vi "AutoSchedule.vi"() -> ()   [LabVIEW 2012]
uses:
  <vilib>/Utility/NIReport.llb/NI_report.lvclass
  <vilib>/addons/database/Auxilliary.llb/DB Tools Cursor Type.ctl
  <vilib>/addons/_office/_exclsub.llb/font.ctl
  <vilib>/addons/_office/excel.llb/Excel Get Data (str).vi
  <vilib>/addons/database/Connection.llb/DB Tools Open Connec (Path).vi
  <vilib>/addons/database/Connection.llb/Conn Execute.vi
  <vilib>/addons/database/Recordset.llb/Rec Fetch Recordset Data (R).vi
  <vilib>/addons/database/Recordset.llb/Rec Destroy - Connection.vi
  <vilib>/Utility/NIReport.llb/Excel/NI_Excel.lvclass
  <vilib>/addons/_office/NI_ReportGenerationToolkit.lvlib
  <vilib>/addons/database/NI_Database_API.lvlib
panel:
  out "error out":errorcluster
  out "concatenated string 2":string
  out "error out 5":errorcluster
  in  "start (0, 0) 4":cluster{"start row":i32, "start column":i32}
  out "concatenated string":string
  in  "start (0, 0) 3":cluster{"start row":i32, "start column":i32}
  out "Numeric":i32
  out "ExcelRow":i32
  in  "start (0, 0)":cluster{"start row":i32, "start column":i32}
  out "x+y":i32
  in  "start (0, 0) 2":cluster{"start row":i32, "start column":i32}
  out "row":i32
  out "array":string[][](array[string])
  out "error out 4":errorcluster
  out "spreadsheet string":string
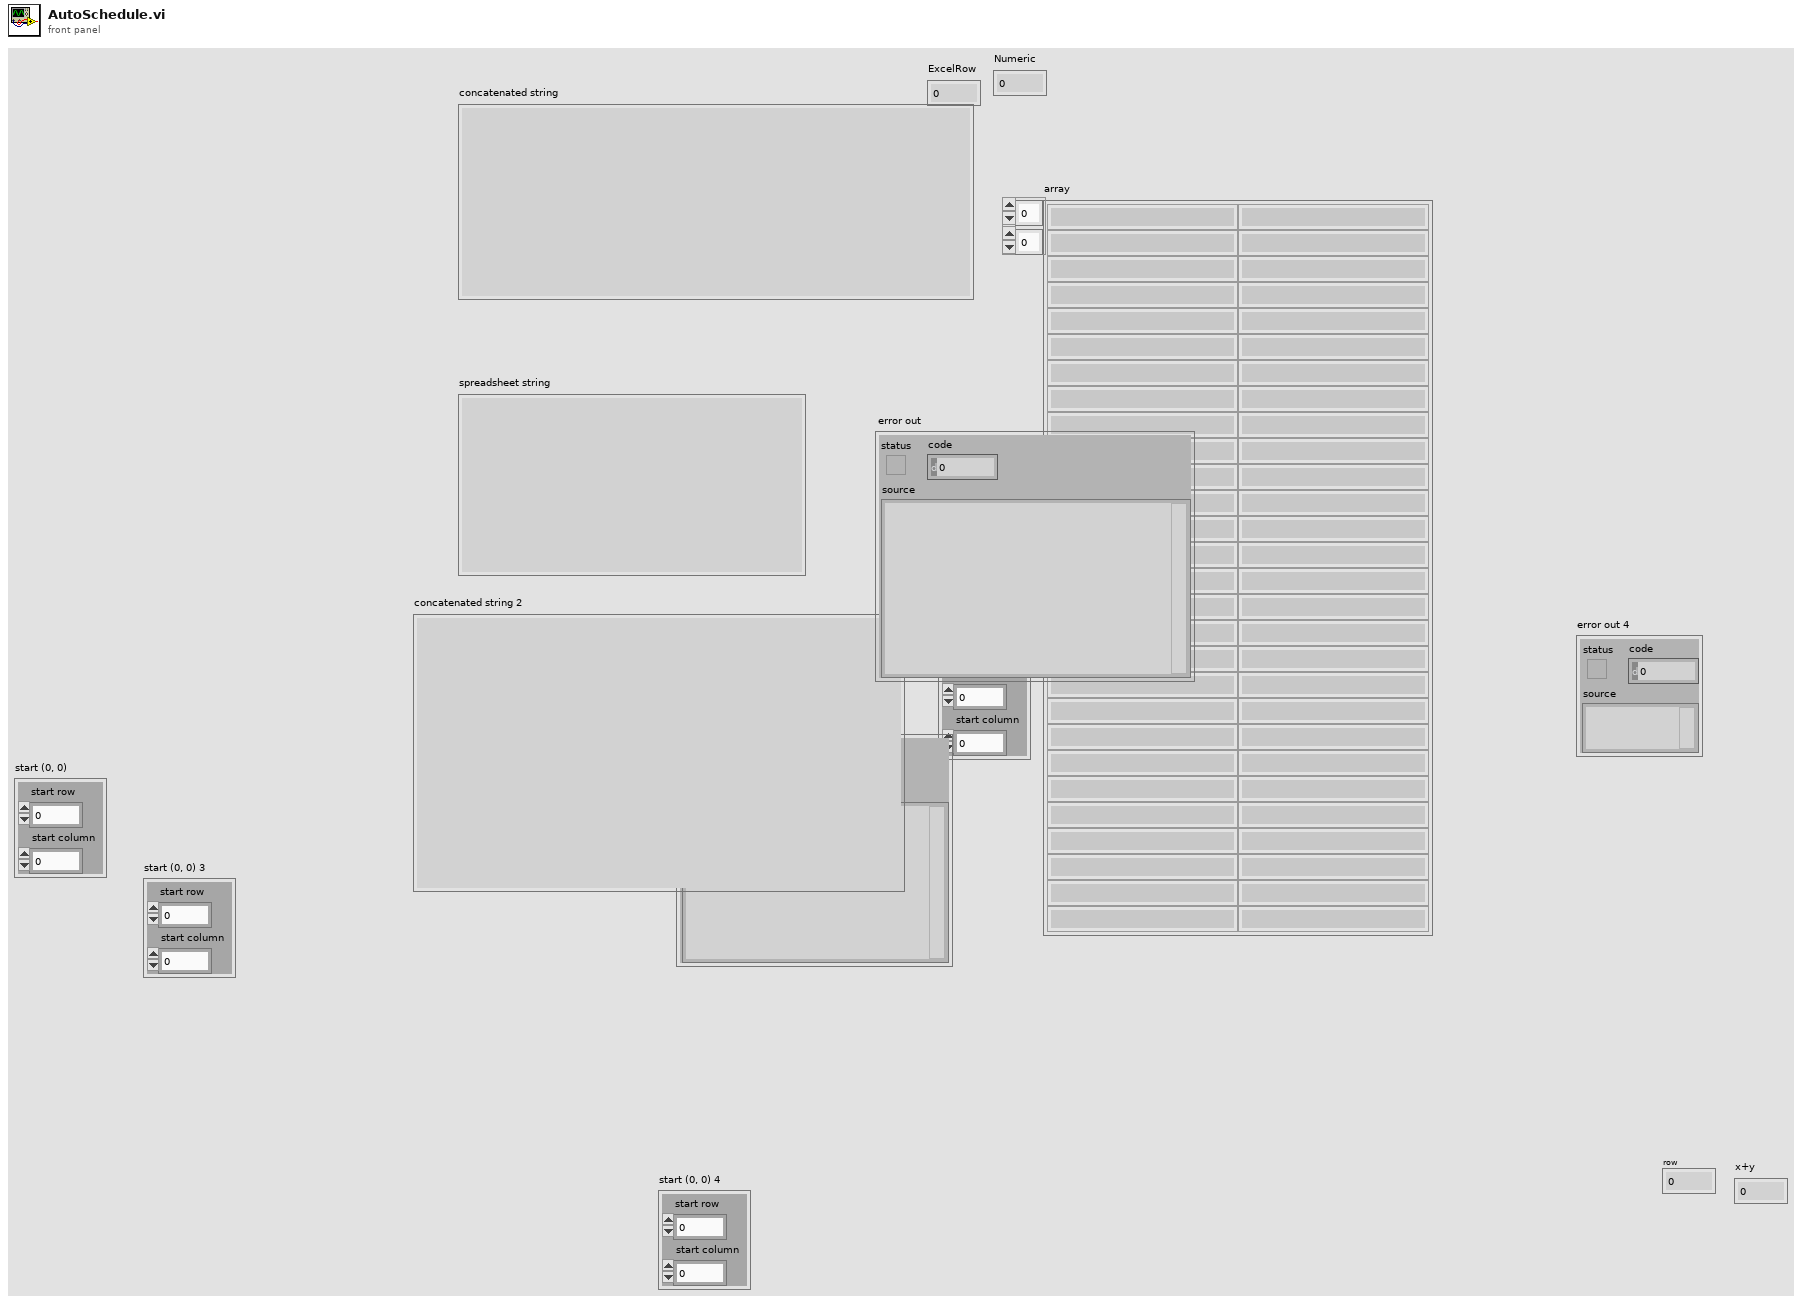
[diagram p1: front panel]
types:
  T1 = enum16{"Standard Report", "HTML", "Word", "Excel"}
  T2 = typedef "NI_ReportGenerationToolkit.lvlib/font.ctl" = cluster{"font name":string, "font size":dbl, "bold":u16, "italic":u16, "underline":u16, "strike through":u16, "font color":u32}
  T3 = cluster{"on/off":bool, "weight":i32, "color":u32}
  T4 = typedef "NI_Database_API.lvlib/DB Tools Cursor Type.ctl" = enum16{"forward-only", "keyset", "dynamic", "static"}
  T5 = typedef "NI_Database_API.lvlib/Conn ObjectReference.ctl" = refnum<k1>
  T6 = typedef "NI_Database_API.lvlib/Rec ObjectReference.ctl" = refnum<k1>
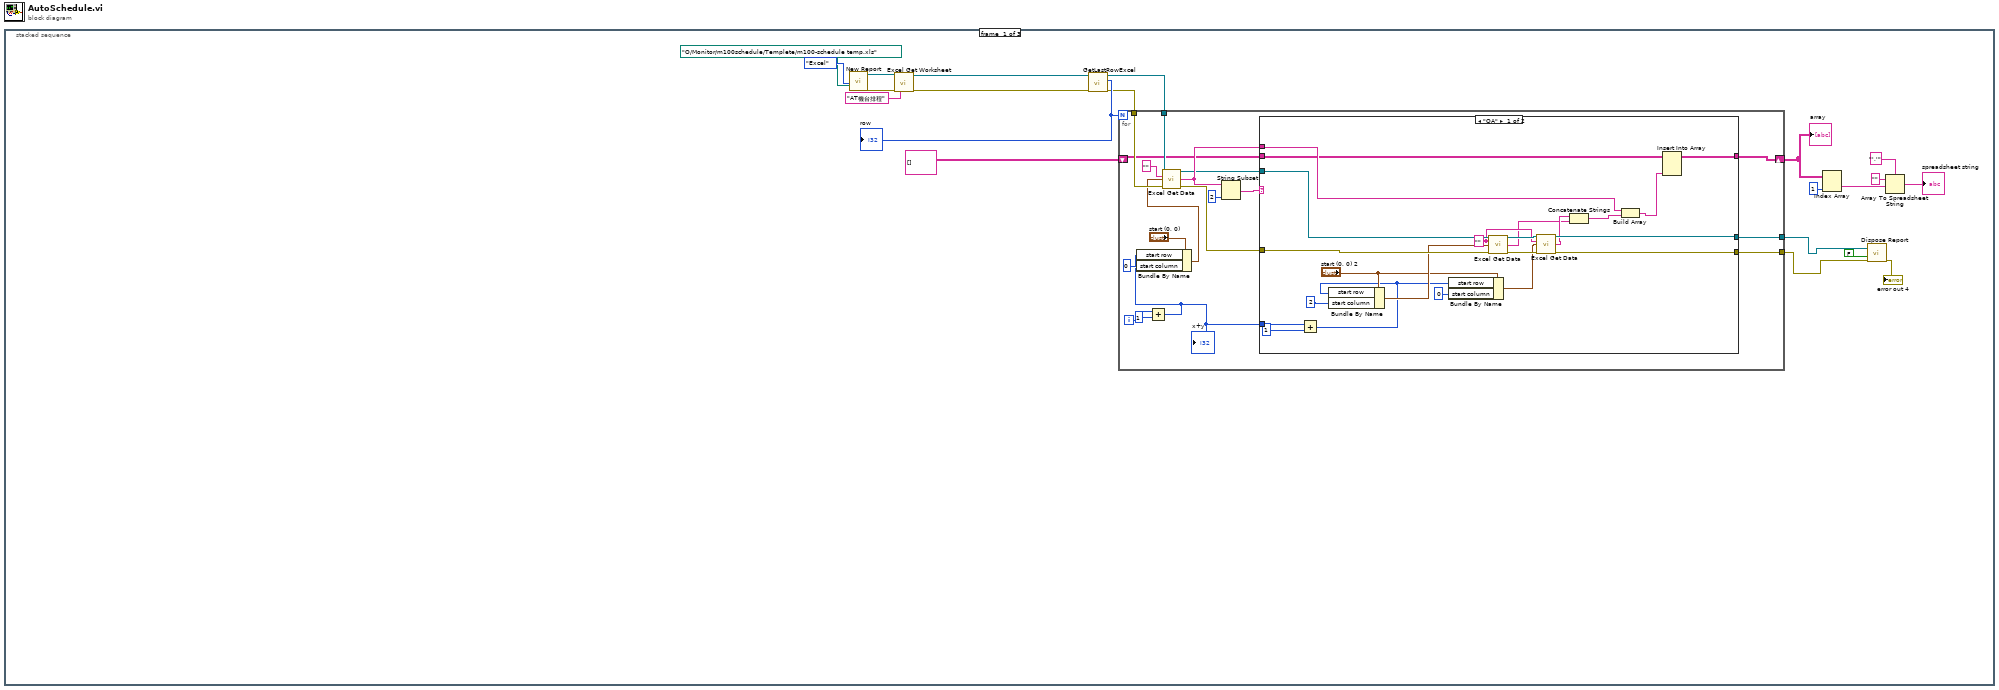
[diagram p0: block diagram]
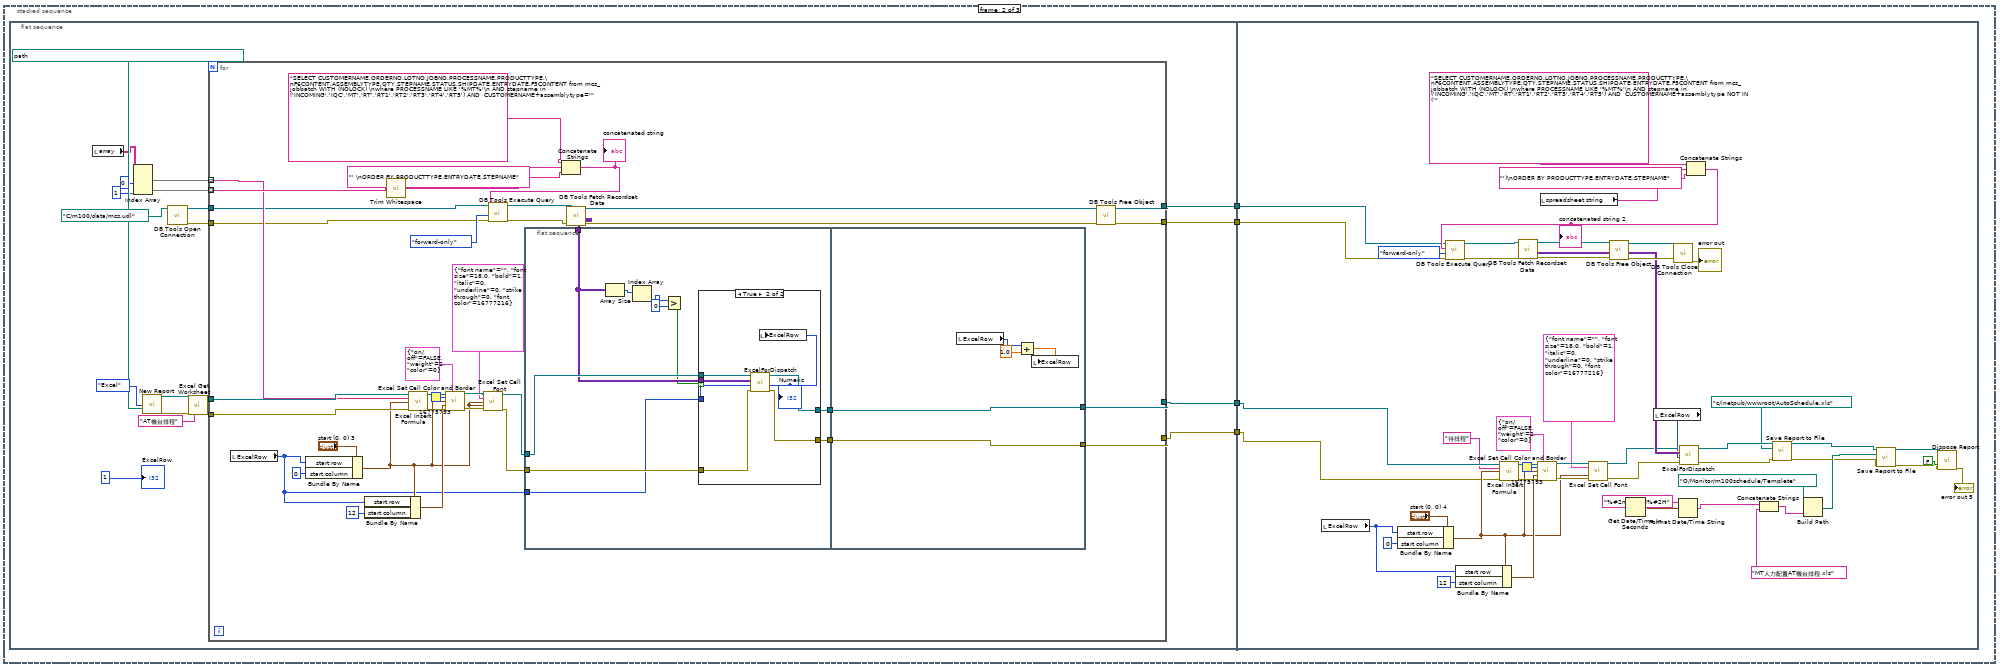
[diagram p3: hidden frame]
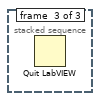
[diagram p5: hidden frame]
diagram:
  n1 = stacked-sequence {
    frame #0 {
      n2 = call <vilib>:"New Report.vi"("report type"=T1."Excel" ("Report Type"), "template (empty)"=path "O:/Monitor/m100schedule/Templete/m100-schedule temp.xls") -> ("report out"=w20:refnum<class "NI_report.lvclass">, "error out"=w19:errorcluster)  [unwired: 12 in]
      n3 = call <vilib>:"Excel Get Worksheet.vi"("report in"=w20, "error in (no error)"=w19, "name (\"\")"="AT機台排程" ("name (\"\")")) -> ("report out"=w18:refnum<class "NI_report.lvclass">, "error out"=w17:errorcluster)  [unwired: 11 in]
      n4 = call "GetLastRowExcel.vi"("error in (no error)"=w17, "report in"=w18) -> ("error out"=w13:errorcluster, "row"=w16:i32, "report out"=w12:refnum<class "NI_report.lvclass">)  [unwired: 7 in]
      "row" <- w16
      n5 = for {
        N: w16 -> [_]
        tunnel: w12 -> [w39]
        tunnel: w13 -> [w38]
        shift-right: [w27] -> w3
        shift-left: string[][] [] ("array") -> [w28]
        tunnel: [w23] -> w8
        tunnel: [w22] -> w7
        i -> [w34]
        n6 = Add(x=w34, y=1) -> (x+y=w24:i32)
        "x+y" <- w24
        n7 = Bundle By Name(cluster="start (0, 0)", "start row"=w24, "start column"=0) -> (w35:cluster{"start row":i32, "start column":i32})
        n8 = call-poly <vilib>:"Excel Get Data.vi"("report in"=w39, "data type"="", "start (0, 0)"=w35, "error in (no error)"=w38) -> ("report out"=w26:refnum<class "NI_report.lvclass">, "data"=w30:string, "error out"=w25:errorcluster)  [unwired: 9 in]
        n9 = String Subset(string=w30, length (rest)=2 ("length (rest)")) -> (substring=w31:string)  [unwired: 1 in]
        n10 = case shown="\"QA\"" w31 {
          tunnel: w30 -> [w61 _]
          tunnel: w28 -> [w58 w64]
          tunnel: [w59 w64] -> w27
          tunnel: w26 -> [w57 w63]
          tunnel: w25 -> [w56 w62]
          tunnel: w24 -> [w53 _]
          tunnel: [w50 w63] -> w23
          tunnel: [w48 w62] -> w22
          frame "QA" {
            w47 = "" ("data type")
            n11 = Add(x=w53, y=1) -> (x+y=w44:i32)
            n12 = Bundle By Name(cluster="start (0, 0) 2", "start row"=w44, "start column"=2) -> (w55:cluster{"start row":i32, "start column":i32})
            n13 = Bundle By Name(cluster="start (0, 0) 2", "start row"=w44, "start column"=0) -> (w46:cluster{"start row":i32, "start column":i32})
            n14 = call-poly <vilib>:"Excel Get Data.vi"("report in"=w57, "data type"=w47, "start (0, 0)"=w55, "error in (no error)"=w56) -> ("report out"=w51:refnum<class "NI_report.lvclass">, "data"=w41:string, "error out"=w49:errorcluster)  [unwired: 9 in]
            n15 = call-poly <vilib>:"Excel Get Data.vi"("report in"=w51, "data type"=w47, "start (0, 0)"=w46, "error in (no error)"=w49) -> ("report out"=w50:refnum<class "NI_report.lvclass">, "data"=w42:string, "error out"=w48:errorcluster)  [unwired: 9 in]
            n16 = Concatenate Strings(w42, w41) -> (w40:string)
            n17 = Build Array(w61, w40) -> (w60:string[])
            n18 = Insert Into Array(array=w58, new element=w60) -> (w59:string[][])  [unwired: 2 in]
          }
          frame Default {
          }
        }
      }
      "array" <- w3
      n19 = Index Array(array=w3, index (col)=1 ("disabled index (col)")) -> (element=w1:string[])  [unwired: 1 in]
      n20 = call-dynamic "Dispose Report.vi"("report in"=w8, "save changes? (F)"=FALSE, "error in (no error)"=w7) -> ("error out"=→"error out 4":errorcluster)  [unwired: 12 in]
      n21 = Array To Spreadsheet String(delimiter (Tab)="','", array=w1, 3:"" ("format string")) -> (spreadsheet string=→"spreadsheet string":string)
    }
    frame #1 {
      n22 = flat-sequence {
        tunnel: [w72] -> w68
        tunnel: [w71] -> w67
        tunnel: [w70] -> w66
        tunnel: [w69] -> w65
        tunnel: w68 -> [w186]
        tunnel: w67 -> [w185]
        tunnel: w66 -> [w157]
        tunnel: w65 -> [w156]
        frame #0 {
          n23 = local read "array"() -> (w83:string[][])
          n24 = Index Array(array=w83, index (col) #1=0 ("disabled index (col)"), index (col) #2=1 ("index (col)")) -> (element #1=w82:string[], element #2=w79:string[])  [unwired: 2 in]
          n25 = call <vilib>:"New Report.vi"("report type"=T1."Excel" ("Report Type"), "template (empty)"=path "O:/Monitor/m100schedule/Templete/MT人力配置AT機台排程.xls" ("template (empty) 2")) -> ("report out"=w87:refnum<class "NI_report.lvclass">, "error out"=w86:errorcluster)  [unwired: 12 in]
          n26 = call-poly <vilib>:"DB Tools Open Connection.vi"("connection information"=path "C:/m100/data/mcs.udl") -> ("error out"=w73:errorcluster, "connection reference"=w74:T5)  [unwired: 7 in]
          n27 = call <vilib>:"Excel Get Worksheet.vi"("report in"=w87, "error in (no error)"=w86, "name (\"\")"="AT機台排程" ("name (\"\")")) -> ("report out"=w78:refnum<class "NI_report.lvclass">, "error out"=w77:errorcluster)  [unwired: 11 in]
          n28 = for {
            tunnel: w82 -> [w112] mode=indexing
            tunnel: w79 -> [w117] mode=indexing
            tunnel: w78 -> [w114]
            tunnel: w77 -> [w113]
            tunnel: [w97] -> w70
            tunnel: [w96] -> w69
            tunnel: w74 -> [w95]
            tunnel: w73 -> [w94]
            tunnel: [w93] -> w72
            tunnel: [w92] -> w71
            n29 = local read "ExcelRow"() -> (w89:i32)
            n30 = Bundle By Name(cluster="start (0, 0) 3", "start row"=w89, "start column"=0) -> (w99:cluster{"start row":i32, "start column":i32})
            n31 = Bundle By Name(cluster=w99, "start row"=w89, "start column"=12) -> (w104:cluster{"start row":i32, "start column":i32})
            n32 = call <vilib>:"Trim Whitespace.vi"("string"=w117) -> ("trimmed string"=w116:string)  [unwired: 1 in]
            n33 = call <vilib>:"Excel Insert Formula.vi"("report in"=w114, "formula"=w112, "start (0, 0)"=w99, "error in (no error)"=w113) -> ("report out"=w109:refnum<class "NI_report.lvclass">, "error out"=w108:errorcluster)  [unwired: 10 in]
            n34 = call <vilib>:"Excel Set Cell Color and Border.vi"("report in"=w109, "inside border"=T3 {"on/off"=FALSE, "weight"=2, "color"=0}, "background color (w)"=u32 16775793, "start (-1, -1)"=w99, "end (-1, -1)"=w104, "error in (no error)"=w108) -> ("report out"=w103:refnum<class "NI_report.lvclass">, "error out"=w102:errorcluster)  [unwired: 8 in]
            n35 = call <vilib>:"Excel Set Cell Font.vi"("report in"=w103, "font"=T2 {"font name"="", "font size"=18.0, "bold"=1, "italic"=0, "underline"=0, "strike through"=0, "font color"=16777216}, "start (-1, -1)"=w99, "end (-1, -1)"=w99, "error in (no error)"=w102) -> ("report out"=w101:refnum<class "NI_report.lvclass">, "error out"=w100:errorcluster)  [unwired: 9 in]
            n36 = flat-sequence {
              tunnel: w115 -> [w130]
              tunnel: w101 -> [w135]
              tunnel: w100 -> [w134]
              tunnel: [w133] -> w91
              tunnel: [w132] -> w90
              tunnel: w89 -> [w131]
              tunnel: [w146] -> w97
              tunnel: w91 -> [w146]
              tunnel: [w145] -> w96
              tunnel: w90 -> [w145]
              frame #0 {
                n37 = Array Size(array=w130) -> (size(s)=w129:i32[])
                n38 = Index Array(array=w129) -> (element=w128:i32)  [unwired: 1 in]
                n39 = Greater?(x=w128, y=0) -> (0:w126:bool)
                n40 = case shown="True" w126 {
                  tunnel: w135 -> [w137 w144]
                  tunnel: w134 -> [w136 w143]
                  tunnel: [w137 w142] -> w133
                  tunnel: [w136 w141] -> w132
                  tunnel: w131 -> [_ w139]
                  tunnel: w130 -> [_ w138]
                  frame False {
                  }
                  frame True {
                    n41 = call "ExcelForDispatch.vi"("error out"=w143, "RowNo"=w139, "array"=w138, "report out"=w144) -> ("error out 2"=w141:errorcluster, "Numeric"=w140:i32, "report out 2"=w142:refnum<class "NI_report.lvclass">)  [unwired: 5 in]
                    "Numeric" <- w140
                    n42 = local write "ExcelRow"(w140) -> ()
                  }
                }
              }
              frame #1 {
                n43 = local read "ExcelRow"() -> (w148:i32)
                n44 = Add(x=w148, y=1.0) -> (x+y=w147:dbl)
                n45 = local write "ExcelRow"(w147) -> ()
              }
            }
            n46 = Concatenate Strings("SELECT CUSTOMERNAME,ORDERNO,LOTNO,JOBNO,PROCESSNAME,PRODUCTTYPE,\nF6CONTENT,ASSEMBLYTYPE,QTY,STEPNAME,STATUS,SHIPDATE,ENTRYDATE,F5CONTENT from mcs_jobbatch WITH (NOLOCK) \nwhere PROCESSNAME LIKE '%MT%'\n AND stepname in ('INCOMING','IQC','MT','RT','RT1','RT2','RT3','RT4','RT5') AND  CUSTOMERNAME+assemblytype='" ("SQL query"), w116, "' \nORDER BY PRODUCTTYPE,ENTRYDATE,STEPNAME" ("string")) -> (w119:string)
            "concatenated string" <- w119
            n47 = call-poly <vilib>:"DB Tools Execute Query.vi"("error in (no error)"=w94, "cursor type"=DB_Tools_Cursor_Type."forward-only", "SQL query"=w119, "connection reference"=w95) -> ("error out"=w123:errorcluster, "recordset reference"=w125:T6)  [unwired: 4 in]
            n48 = call-poly <vilib>:"DB Tools Fetch Recordset Data.vi"("error in (no error)"=w123, "recordset reference"=w125) -> ("error out"=w122:errorcluster, "recordset data"=w115:variant[][], "recordset reference out"=w124:T6)  [unwired: 3 in]
            n49 = call-poly <vilib>:"DB Tools Free Object.vi"("error in (no error)"=w122, "recordset reference"=w124) -> ("error out"=w92:errorcluster, "connection reference"=w93:T5)  [unwired: 8 in]
          }
          "ExcelRow" <- 1
        }
        frame #1 {
          n50 = local read "ExcelRow"() -> (w160:i32)
          n51 = Bundle By Name(cluster="start (0, 0) 4", "start row"=w160, "start column"=0) -> (w162:cluster{"start row":i32, "start column":i32})
          n52 = Bundle By Name(cluster=w162, "start row"=w160, "start column"=12) -> (w165:cluster{"start row":i32, "start column":i32})
          n53 = call <vilib>:"Excel Insert Formula.vi"("report in"=w157, "formula"="待排程", "start (0, 0)"=w162, "error in (no error)"=w156) -> ("report out"=w170:refnum<class "NI_report.lvclass">, "error out"=w169:errorcluster)  [unwired: 10 in]
          n54 = call <vilib>:"Excel Set Cell Color and Border.vi"("report in"=w170, "inside border"=T3 {"on/off"=FALSE, "weight"=2, "color"=0}, "background color (w)"=u32 16775793, "start (-1, -1)"=w162, "end (-1, -1)"=w165, "error in (no error)"=w169) -> ("report out"=w164:refnum<class "NI_report.lvclass">, "error out"=w163:errorcluster)  [unwired: 8 in]
          n55 = local read "spreadsheet string"() -> (w191:string)
          n56 = call <vilib>:"Excel Set Cell Font.vi"("report in"=w164, "font"=T2 {"font name"="", "font size"=18.0, "bold"=1, "italic"=0, "underline"=0, "strike through"=0, "font color"=16777216}, "start (-1, -1)"=w162, "end (-1, -1)"=w162, "error in (no error)"=w163) -> ("report out"=w159:refnum<class "NI_report.lvclass">, "error out"=w158:errorcluster)  [unwired: 9 in]
          n57 = Get Date/Time In Seconds() -> (seconds since 1Jan1904=w175:timestamp)
          n58 = local read "ExcelRow"() -> (w187:i32)
          n59 = Format Date/Time String(time format string (%c)="%#2m%#2d%#2H", seconds (now)=w175) -> (date/time string=w173:string)  [unwired: 1 in]
          n60 = Concatenate Strings("SELECT CUSTOMERNAME,ORDERNO,LOTNO,JOBNO,PROCESSNAME,PRODUCTTYPE,\nF6CONTENT,ASSEMBLYTYPE,QTY,STEPNAME,STATUS,SHIPDATE,ENTRYDATE,F5CONTENT from mcs_jobbatch WITH (NOLOCK) \nwhere PROCESSNAME LIKE '%MT%'\n AND stepname in ('INCOMING','IQC','MT','RT','RT1','RT2','RT3','RT4','RT5') AND  CUSTOMERNAME+assemblytype NOT IN ('" ("SQL query"), w191, "')\nORDER BY PRODUCTTYPE,ENTRYDATE,STEPNAME" ("string")) -> (w189:string)
          "concatenated string 2" <- w189
          n61 = call-poly <vilib>:"DB Tools Execute Query.vi"("error in (no error)"=w185, "cursor type"=DB_Tools_Cursor_Type."forward-only", "SQL query"=w189, "connection reference"=w186) -> ("error out"=w197:errorcluster, "recordset reference"=w199:T6)  [unwired: 4 in]
          n62 = call-poly <vilib>:"DB Tools Fetch Recordset Data.vi"("error in (no error)"=w197, "recordset reference"=w199) -> ("error out"=w196:errorcluster, "recordset data"=w188:variant[][], "recordset reference out"=w198:T6)  [unwired: 3 in]
          n63 = call-poly <vilib>:"DB Tools Free Object.vi"("error in (no error)"=w196, "recordset reference"=w198) -> ("error out"=w195:errorcluster, "connection reference"=w194:T5)  [unwired: 8 in]
          n64 = call <vilib>:"DB Tools Close Connection.vi"("error in (no error)"=w195, "connection reference"=w194) -> ("error out"=→"error out":errorcluster)  [unwired: 5 in]
          n65 = call "ExcelForDispatch.vi"("error out"=w158, "RowNo"=w187, "array"=w188, "report out"=w159) -> ("error out 2"=w153:errorcluster, "report out 2"=w154:refnum<class "NI_report.lvclass">)  [unwired: 5 in, 1 out]
          n66 = Concatenate Strings(w173, "MT人力配置AT機台排程.xls" ("string")) -> (w177:string)
          n67 = call-dynamic "Save Report to File.vi"("report in"=w154, "report file path"=path "c:/inetpub/wwwroot/AutoSchedule.xls", "error in (no error)"=w153) -> ("report out"=w152:refnum<class "NI_report.lvclass">, "error out"=w151:errorcluster)  [unwired: 11 in]
          n68 = Build Path(base path=path "O:/Monitor/m100schedule/Templete", name or relative path=w177) -> (appended path=w178:path)
          n69 = call-dynamic "Save Report to File.vi"("report in"=w152, "report file path"=w178, "error in (no error)"=w151) -> ("report out"=w180:refnum<class "NI_report.lvclass">, "error out"=w179:errorcluster)  [unwired: 11 in]
          n70 = call-dynamic "Dispose Report.vi"("report in"=w180, "save changes? (F)"=FALSE, "error in (no error)"=w179) -> ("error out"=→"error out 5":errorcluster)  [unwired: 12 in]
        }
      }
    }
    frame #2 {
      n71 = Quit LabVIEW() -> ()  [unwired: 1 in]
    }
  }
